vi "VALVE_main.vi"   [LabVIEW 2015]
uses:
  CONTROLS/Q_main_element.ctl
  CONTROLS/Q_VALVE_element.ctl
  GLOBAL/Global_VALVE.vi
  GLOBAL/Global_ABORT.vi
  GLOBAL/Global_MAIN.vi
types:
  T1 = typedef "Q_VALVE_element.ctl" = cluster{"variant":variant, "Instruction":enum16{"VALVE_idle", "VALVE_initialize", "VALVE_error", "VALVE_security_stop", "VALVE_change_position", "VALVE_two_way_valves", "VALVE_init_merFISH", "VALVE_stop"}}
  T2 = typedef "Q_main_element.ctl" = cluster{"variant":variant, "Instruction":enum16{"Main_idle", "Main_initialize", "Main_initialize_TDMS", "Main_initialize_Queue", "Main_error", "Main_DAQ_initialization_results", "Main_ASI_initialization_results", "Main_Piezo_initialization_results", "Main_Valve_initialization_results", "Main_Pump_initialization_results", "Main_CAMERA_initialization_results", "Main_FPGA_initialization_results", "Main_DAQ_error", "Main_ASI_error", "Main_Piezo_error", "Main_CAMERA_error", "Main_Valve_error", "Main_Pump_error", "Main_FPGA_error", "Main_start_acquiring", "Main_not_acquiring", "Main_acquiring", "Main_stop_acquiring", "Main_change_exposure", "Main_change_z_scan_parameters", "Main_define_ROI", "Main_define_mosaic", "Main_read_kinetic_time", "Main_cooler", "Main_read_temperature", "Main_save_XY", "Main_load_XY", "Main_discard_XY", "Main_move_to_XY", "Main_measure_QPD", "Main_autofocus_calibration", "Main_autofocus_initialization", "Main_autofocus_stop", "Main_save_PID", "Main_change_H_valve_position", "Main_two_way_valve", "Main_save_movie", "Main_init_single_scan", "Main_single_scan", "Main_stop_single_scan", "Main_merFISH_illumination_parameters", "Main_merFISH_buffer_probe_list", "Main_merFISH_injections_procedure", "Main_merFISH_save_setpoint", "Main_merFISH_DAPI_parameters", "Main_merFISH_Brightfield_parameters", "Main_merFISH_save_embryo_ROI", "Main_merFISH_init", "Main_merFISH_resume", "Main_merFISH_start_autofocus", "Main_merFISH_open_close_valve_merFISH", "Main_merFISH_open_close_valve_photobleaching", "Main_merFISH_hybridization", "Main_merFISH_move_to_ROI", "Main_merFISH_wait_stabilization", "Main_merFISH_move_to_REF", "Main_merFISH_scan", "Main_merFISH_photobleaching_injection", "Main_merFISH_photobleaching", "Main_merFISH_send_email", "Main_merFISH_close", "Main_STOP"}}
  T3 = enum16{"VALVE_idle", "VALVE_initialize", "VALVE_error", "VALVE_security_stop", "VALVE_change_position", "VALVE_two_way_valves", "VALVE_init_merFISH", "VALVE_stop"}
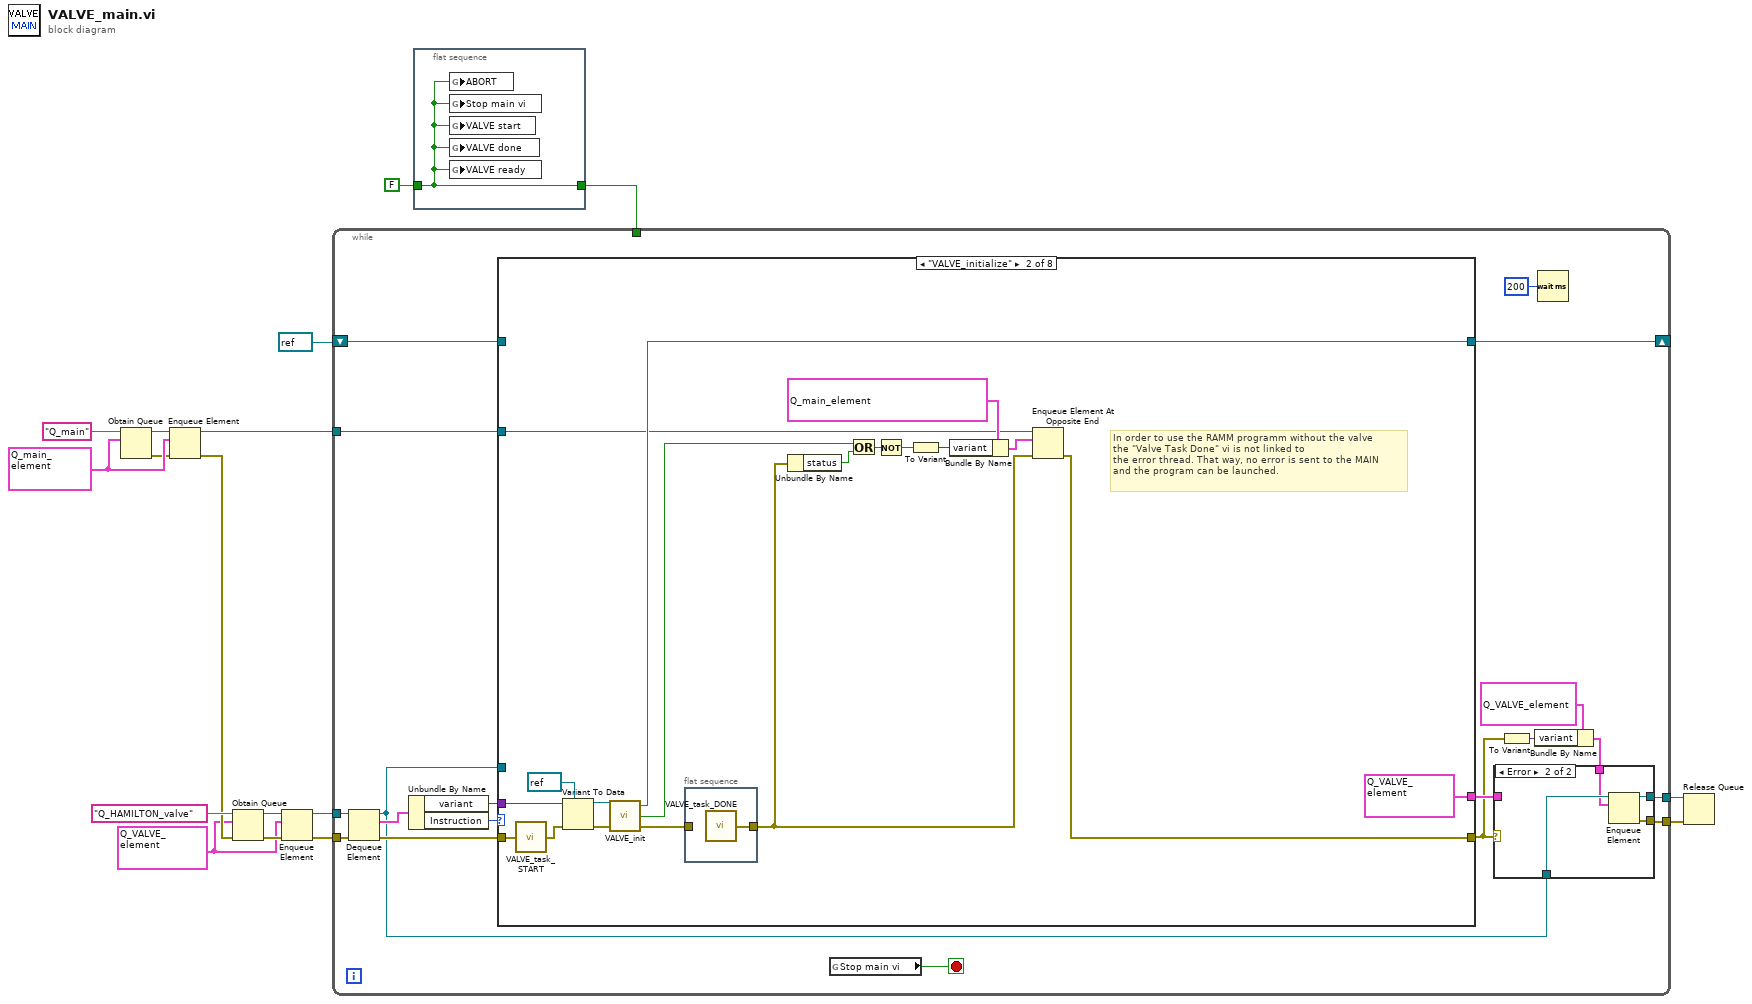
[diagram p0: block diagram]
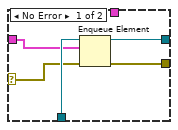
[diagram p2: hidden frame]
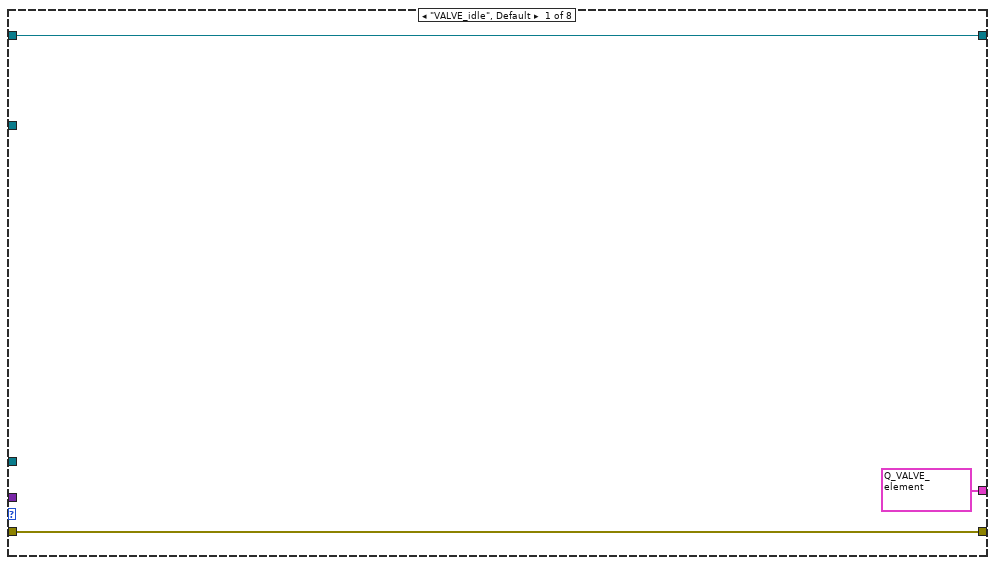
[diagram p3: hidden frame]
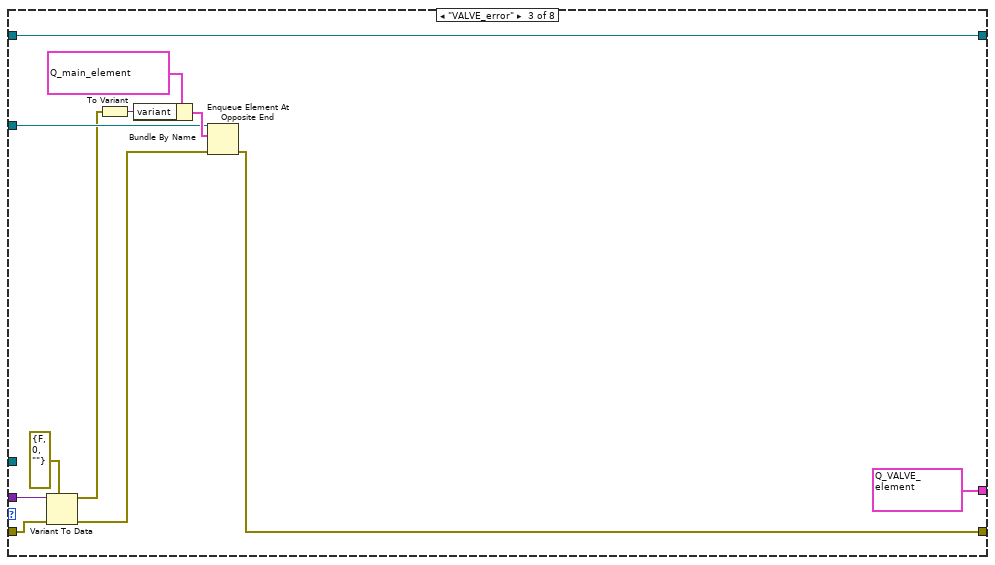
[diagram p4: hidden frame]
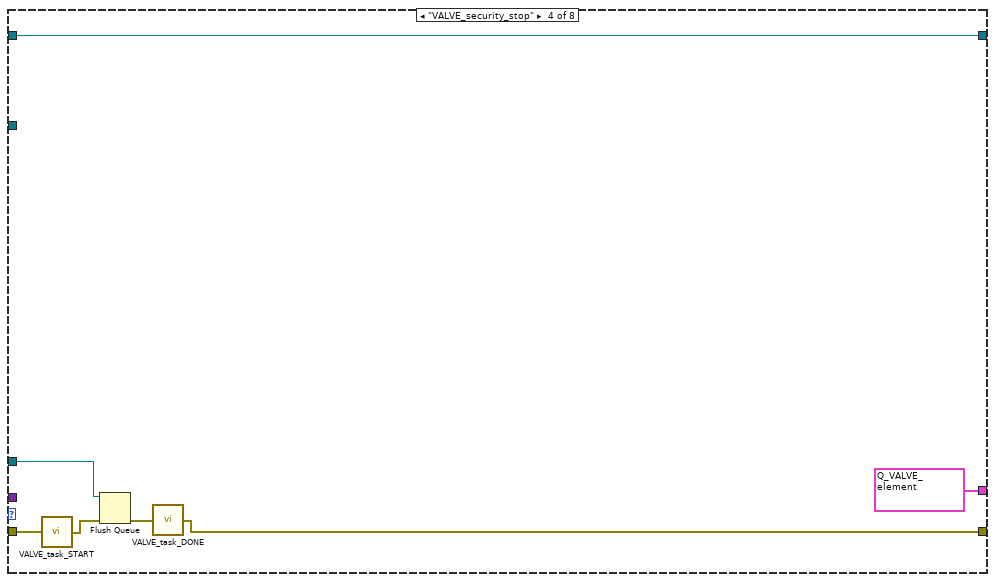
[diagram p5: hidden frame]
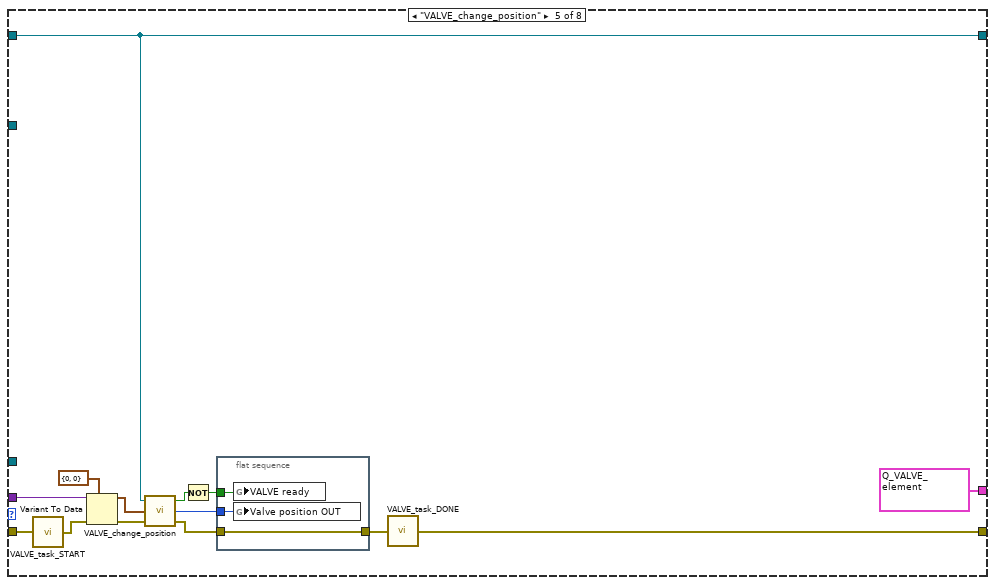
[diagram p6: hidden frame]
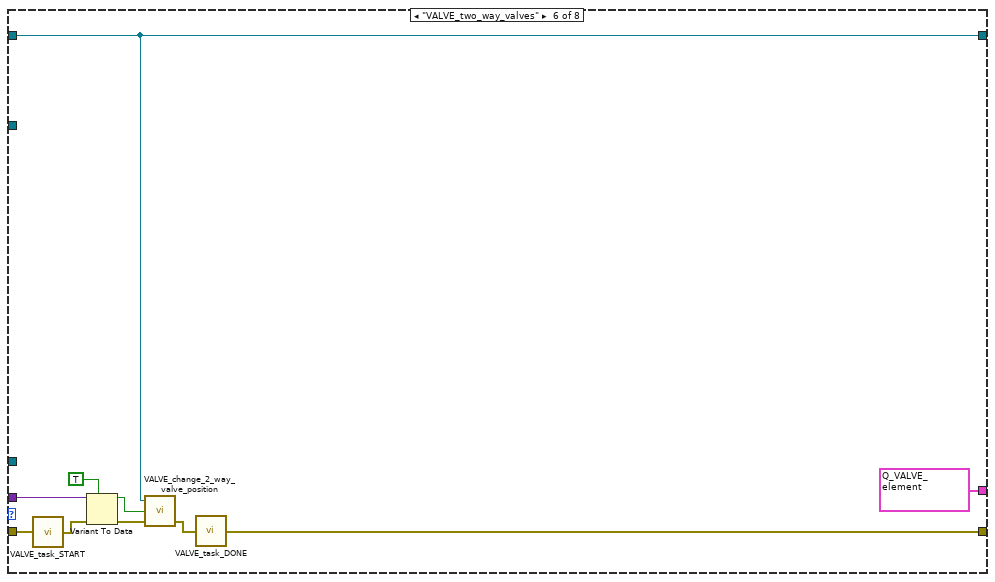
[diagram p7: hidden frame]
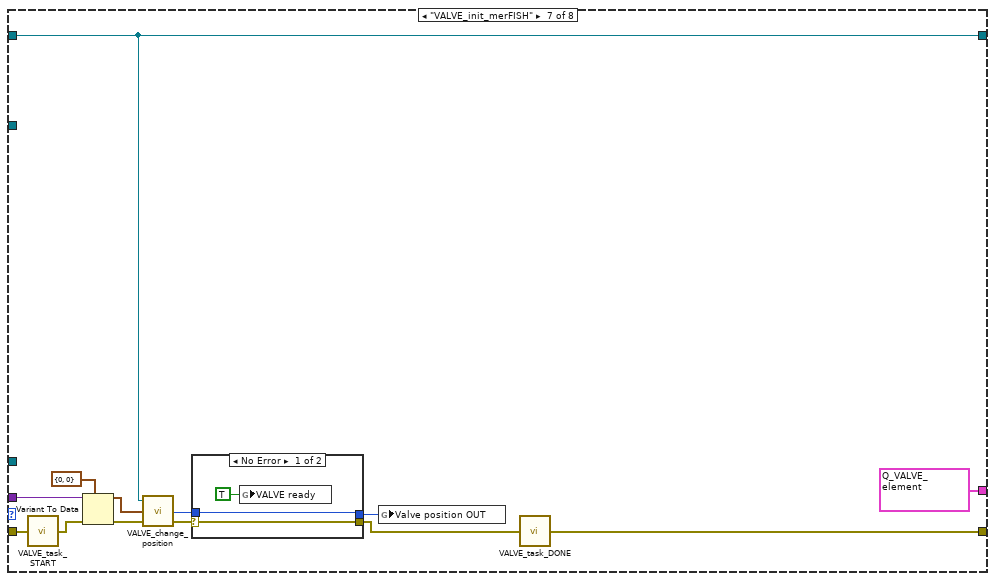
[diagram p8: hidden frame]
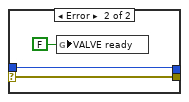
[diagram p9: hidden frame]
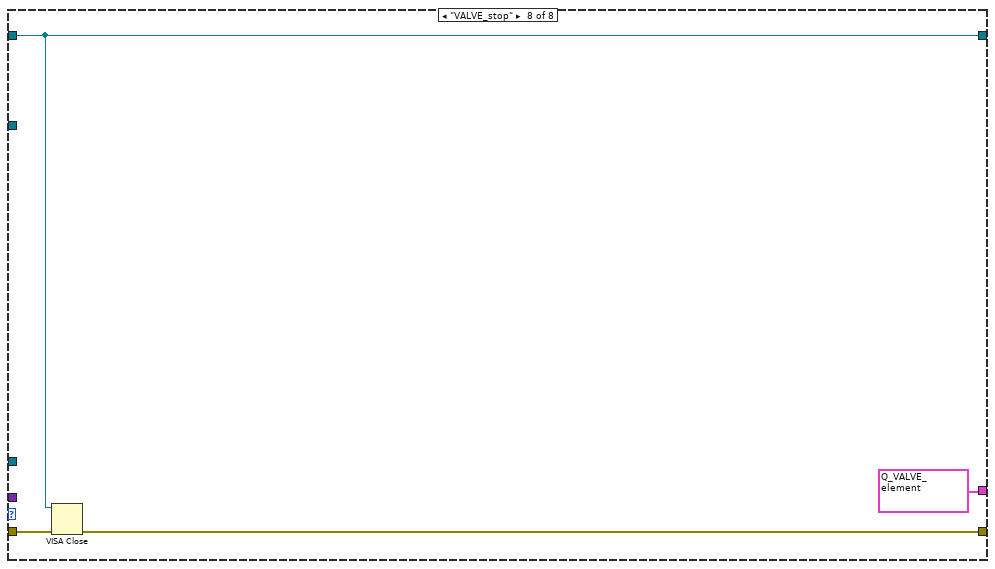
[diagram p10: hidden frame]
diagram:
  w2 = T1 {"variant"=variant, "Instruction"=enum."VALVE_idle"} ("Q_VALVE")
  w10 = T2 {"variant"=variant, "Instruction"=enum."Main_idle"} ("Q_main_element")
  n1 = Obtain Queue(name (unnamed)="Q_main", element data type=w10) -> (queue out=w8:refnum<queue>, error out=w9:errorcluster)  [unwired: 3 in, 1 out]
  n2 = Enqueue Element(queue=w8, element=w10, error in (no error)=w9) -> (queue out=w6:refnum<queue>, error out=w3:errorcluster)  [unwired: 1 in, 1 out]
  n3 = Obtain Queue(name (unnamed)="Q_HAMILTON_valve", element data type=w2, error in (no error)=w3) -> (queue out=w16:refnum<queue>, error out=w15:errorcluster)  [unwired: 2 in, 1 out]
  n4 = Enqueue Element(queue=w16, element=w2, error in (no error)=w15) -> (queue out=w14:refnum<queue>, error out=w13:errorcluster)  [unwired: 1 in, 1 out]
  n5 = while {
    tunnel: w14 -> [w35]
    tunnel: w13 -> [w34]
    tunnel: [w29] -> w12
    tunnel: [w28] -> w11
    tunnel: w6 -> [w27]
    tunnel: w4 -> [_]
    shift-right: [w19] -> _
    shift-left: refnum<visa-resource-name> refnum ("VISA resource name out") -> [w20]
    stop <- w36 stop-if-true
    n6 = Dequeue Element(queue=w35, error in (no error)=w34) -> (queue out=w18:refnum<queue>, element=w33:T1, error out=w31:errorcluster)  [unwired: 1 in, 1 out]
    n7 = Unbundle By Name(w33) -> ("variant"=w26:variant, "Instruction"=w32:T3)
    n8 = case shown="\"VALVE_initialize\"" w32 {
      tunnel: w31 -> [w48 w67 w77 w85 w96 w111 w127 w136]
      tunnel: [w48 w54 w69 w81 w90 w109 w117 w134] -> w23
      tunnel: [T1 {"variant"=variant, "Instruction"=enum."VALVE_idle"} ("Q_VALVE") T1 {"variant"=variant, "Instruction"=enum."VALVE_idle"} ("Q_VALVE") T1 {"variant"=variant, "Instruction"=enum."VALVE_idle"} ("Q_VALVE") T1 {"variant"=variant, "Instruction"=enum."VALVE_idle"} ("Q_VALVE") T1 {"variant"=variant, "Instruction"=enum."VALVE_idle"} ("Q_VALVE") T1 {"variant"=variant, "Instruction"=enum."VALVE_idle"} ("Q_VALVE") T1 {"variant"=variant, "Instruction"=enum."VALVE_idle"} ("Q_VALVE") T1 {"variant"=variant, "Instruction"=enum."VALVE_idle"} ("Q_VALVE")] -> w30
      tunnel: w27 -> [_ w56 w72 _ _ _ _ _]
      tunnel: w26 -> [_ w65 w78 _ w101 w114 w126 _]
      tunnel: w18 -> [_ _ _ w83 _ _ _ _]
      tunnel: w20 -> [w46 _ w79 w86 w97 w112 w124 w135]
      tunnel: [w46 w60 w79 w86 w97 w112 w124 w135] -> w19
      frame "VALVE_idle", Default {
      }
      frame "VALVE_initialize" {
        # "In order to use the RAMM programm without the valve \nthe \"Valve Task Done\" vi is not linked to \nthe error thread. That way, no error is sent to the MAIN \nand the program can be launched."
        n9 = call "VALVE_task_START.vi"("error in"=w67) -> ("error out"=w64:errorcluster)
        n10 = Variant To Data(error in=w64, type=refnum<visa-resource-name> refnum ("VISA resource name out"), Variant=w65) -> (data=w62:refnum<visa-resource-name>, error out=w63:errorcluster)
        n11 = call "VALVE_init.vi"("error in"=w63, "VISA resource Valve"=w62) -> ("error out"=w49:errorcluster, "Error valve"=w51:bool, "VISA resource name out"=w60:refnum<visa-resource-name>)  [unwired: 1 in]
        n12 = flat-sequence {
          tunnel: [w68] -> w50
          tunnel: w49 -> [_]
          frame #0 {
            n13 = call "VALVE_task_DONE.vi"() -> ("error out"=w68:errorcluster)  [unwired: 1 in]
          }
        }
        n14 = Unbundle By Name(w50) -> ("status"=w52:bool)
        n15 = Or(x=w51, y=w52) -> (x .or. y?=w53:bool)
        n16 = Not(x=w53) -> (.not. x?=w55:bool)
        n17 = To Variant(anything=w55) -> (Variant=w58:variant)
        n18 = Bundle By Name(cluster=T2 {"variant"=variant, "Instruction"=enum."Main_Valve_initialization_results"} ("element"), "variant"=w58) -> (w57:T2)
        n19 = Enqueue Element At Opposite End(queue=w56, element=w57, error in (no error)=w50) -> (error out=w54:errorcluster)  [unwired: 1 in, 2 out]
      }
      frame "VALVE_error" {
        n20 = Variant To Data(error in=w77, type=errorcluster {"status"=FALSE, "code"=0, "source"=""} ("error out"), Variant=w78) -> (data=w71:errorcluster, error out=w70:errorcluster)
        n21 = To Variant(anything=w71) -> (Variant=w74:variant)
        n22 = Bundle By Name(cluster=T2 {"variant"=variant, "Instruction"=enum."Main_Valve_error"} ("Q_main_element"), "variant"=w74) -> (w75:T2)
        n23 = Enqueue Element At Opposite End(queue=w72, element=w75, error in (no error)=w70) -> (error out=w69:errorcluster)  [unwired: 1 in, 2 out]
      }
      frame "VALVE_security_stop" {
        n24 = call "VALVE_task_START.vi"("error in"=w85) -> ("error out"=w84:errorcluster)
        n25 = Flush Queue(queue=w83, error in (no error)=w84) -> (error out=w82:errorcluster)  [unwired: 2 out]
        n26 = call "VALVE_task_DONE.vi"("error in"=w82) -> ("error out"=w81:errorcluster)
      }
      frame "VALVE_change_position" {
        n27 = call "VALVE_task_START.vi"("error in"=w96) -> ("error out"=w95:errorcluster)
        n28 = Variant To Data(error in=w95, type=cluster{"Valve H":u8, "OldVal":u8} {"Valve H"=0, "OldVal"=0} ("output cluster"), Variant=w101) -> (data=w98:cluster{"Valve H":u8, "OldVal":u8}, error out=w99:errorcluster)
        n29 = call "VALVE_change_position.vi"("error in"=w99, "valve positions"=w98, "VISA valve"=w97) -> ("error out"=w94:errorcluster, "Valve position OUT"=w93:u8, "Valve error"=w92:bool)
        n30 = Not(x=w92) -> (.not. x?=w88:bool)
        n31 = flat-sequence {
          tunnel: w94 -> [w103]
          tunnel: w93 -> [w104]
          tunnel: w88 -> [w102]
          tunnel: [w103] -> w91
          frame #0 {
            n32 = global write "Global_VALVE.vi" "VALVE ready"(w102) -> ()
            n33 = global write "Global_VALVE.vi" "Valve position OUT"(w104) -> ()
          }
        }
        n34 = call "VALVE_task_DONE.vi"("error in"=w91) -> ("error out"=w90:errorcluster)
      }
      frame "VALVE_two_way_valves" {
        n35 = call "VALVE_task_START.vi"("error in"=w111) -> ("error out"=w110:errorcluster)
        n36 = Variant To Data(error in=w110, type=TRUE, Variant=w114) -> (data=w106:bool, error out=w113:errorcluster)
        n37 = call "VALVE_change_2_way_valve_position.vi"("error in"=w113, "Valve position"=w106, "VISA valve"=w112) -> ("error out"=w105:errorcluster)  [unwired: 1 in, 1 out]
        n38 = call "VALVE_task_DONE.vi"("error in"=w105) -> ("error out"=w109:errorcluster)
      }
      frame "VALVE_init_merFISH" {
        n39 = call "VALVE_task_START.vi"("error in"=w127) -> ("error out"=w125:errorcluster)
        n40 = Variant To Data(error in=w125, type=cluster{"Valve H":u8, "OldVal":u8} {"Valve H"=0, "OldVal"=0} ("valve positions"), Variant=w126) -> (data=w121:cluster{"Valve H":u8, "OldVal":u8}, error out=w123:errorcluster)
        n41 = call "VALVE_change_position.vi"("error in"=w123, "valve positions"=w121, "VISA valve"=w124) -> ("error out"=w120:errorcluster, "Valve position OUT"=w119:u8)  [unwired: 1 out]
        n42 = case shown="No Error" w120 {
          selector: w120 -> [w128 w132]
          tunnel: [w128 w132] -> w116
          tunnel: [w129 w131] -> w118
          tunnel: w119 -> [w129 w131]
          frame No Error {
            n43 = global write "Global_VALVE.vi" "VALVE ready"(TRUE ("VALVE ready")) -> ()
          }
          frame Error {
            n44 = global write "Global_VALVE.vi" "VALVE ready"(FALSE ("VALVE ready")) -> ()
          }
        }
        n45 = global write "Global_VALVE.vi" "Valve position OUT"(w118) -> ()
        n46 = call "VALVE_task_DONE.vi"("error in"=w116) -> ("error out"=w117:errorcluster)
      }
      frame "VALVE_stop" {
        n47 = VISA Close(VISA resource name=w135, error in (no error)=w136) -> (error out=w134:errorcluster)
      }
    }
    n48 = global read "Global_MAIN.vi" "Stop main vi"() -> (w36:bool)
    n49 = To Variant(anything=w23) -> (Variant=w24:variant)
    n50 = Bundle By Name(cluster=T1 {"variant"=variant, "Instruction"=enum."VALVE_error"} ("Q_VALVE"), "variant"=w24) -> (w25:T1)
    n51 = case shown="Error" w23 {
      selector: w23 -> [w38 _]
      tunnel: w30 -> [w37 _]
      tunnel: [w41 w45] -> w29
      tunnel: [w40 w44] -> w28
      tunnel: w18 -> [w39 w43]
      tunnel: w25 -> [_ w42]
      frame No Error {
        n52 = Enqueue Element(queue=w39, element=w37, error in (no error)=w38) -> (queue out=w41:refnum<queue>, error out=w40:errorcluster)  [unwired: 1 in, 1 out]
      }
      frame Error {
        n53 = Enqueue Element(queue=w43, element=w42) -> (queue out=w45:refnum<queue>, error out=w44:errorcluster)  [unwired: 2 in, 1 out]
      }
    }
    n54 = Wait (ms)(milliseconds to wait=u32 200) -> ()  [unwired: 1 out]
  }
  n55 = flat-sequence {
    tunnel: FALSE ("Stop main vi") -> [w138]
    tunnel: [w138] -> w4
    frame #0 {
      n56 = global write "Global_ABORT.vi" "ABORT"(w138) -> ()
      n57 = global write "Global_MAIN.vi" "Stop main vi"(w138) -> ()
      n58 = global write "Global_VALVE.vi" "VALVE start"(w138) -> ()
      n59 = global write "Global_VALVE.vi" "VALVE done"(w138) -> ()
      n60 = global write "Global_VALVE.vi" "VALVE ready"(w138) -> ()
    }
  }
  n61 = Release Queue(queue=w12, error in (no error)=w11) -> ()  [unwired: 1 in, 3 out]
